vi "writeFile RawTestHead.vi"(8 "Name Array":string[](array[string])=["Wafer name", "Scribe", "Mask", "Lot", "Device name", "Active Area", "Mesa Area", "x", "y", "Imeas", "Vmeas", "Time", "Vset", "Icomp", "Jset", "Iset", "Vcomp", "Laser Power", "TestID", "SessionTime", "Operator"], 11 "Path":path) -> (3 "Path out":path)   [LabVIEW 2012]
uses:
  <vilib>/Utility/file.llb/Write To Spreadsheet File (string).vi
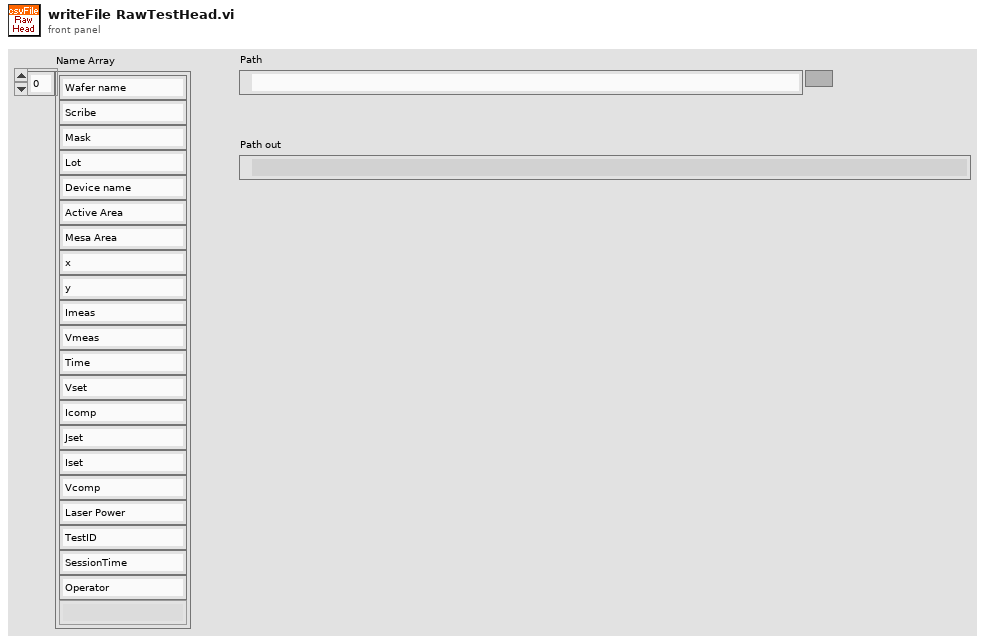
[diagram p1: front panel]
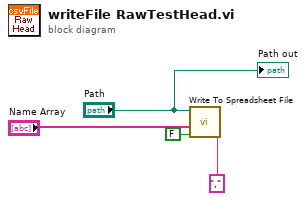
[diagram p0: block diagram]
diagram:
  n1 = call-poly <vilib>:"Write To Spreadsheet File.vi"("delimiter (\\t)"="," ("delimiter (\\t)"), "append to file? (new file:F)"=FALSE, "1D data"="Name Array", "file path (dialog if empty)"="Path") -> ()  [unwired: 4 in, 1 out]
  "Path out" <- "Path"
